vi "Select Physical Channels_Variable.vi"(8 "error in":errorcluster, 11 "Physical Channels In":bool[](array[boolean])) -> (0 "error out":errorcluster, 2 "Cancelled?":bool, 3 "Physical Channels Out":bool[](array[boolean]))   [LabVIEW 2020, in "Waveform Analog Output System Explorer.lvlib"]
doc: "When called, launches a dialogue to select AO channels to be added to the system definition"
uses:
  Waveform Analog Output System Explorer.lvlib
panel:
  in  "Tree":string(tree)
  in  "Cancel":bool
  in  "Accept":bool
  # "Please Select the Channels to Use"
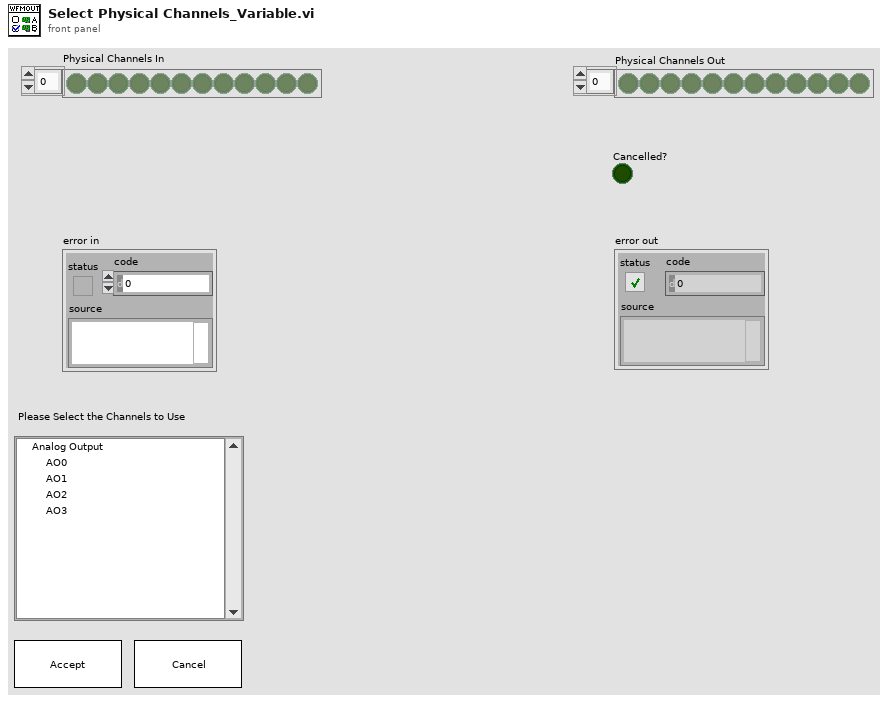
[diagram p1: front panel]
types:
  T1 = typedef "LVPoint32TypeDef.ctl" = cluster{"Horizontal":i32, "Vertical":i32}
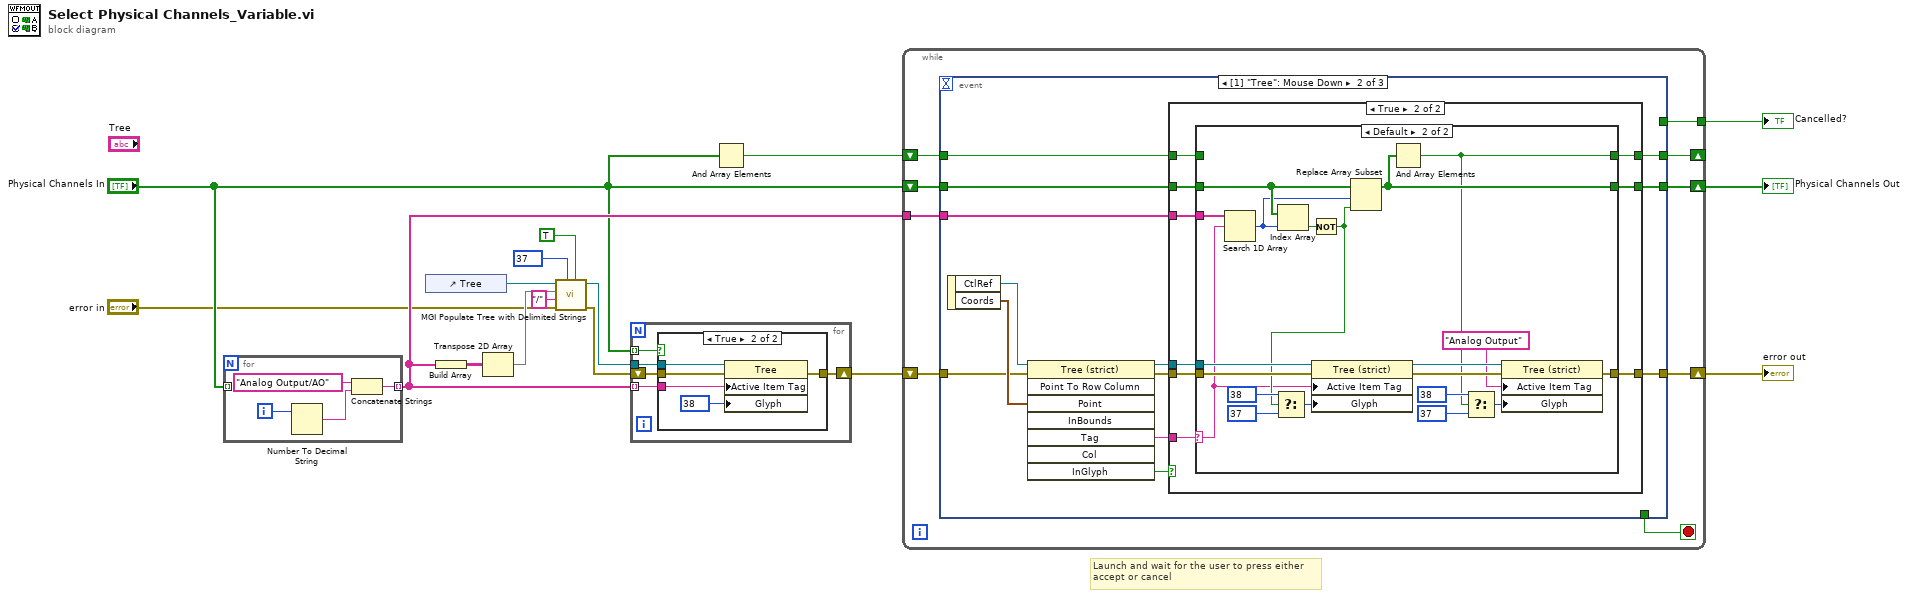
[diagram p0: block diagram]
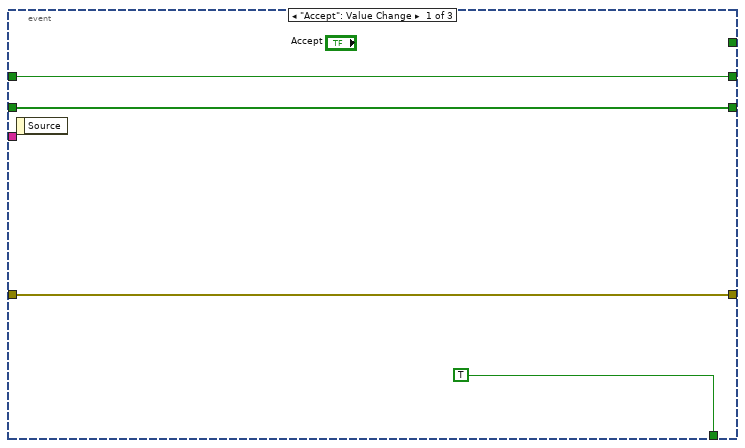
[diagram p3: hidden frame]
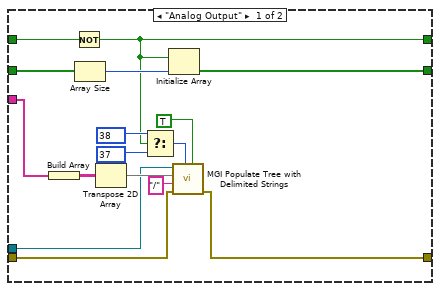
[diagram p5: hidden frame]
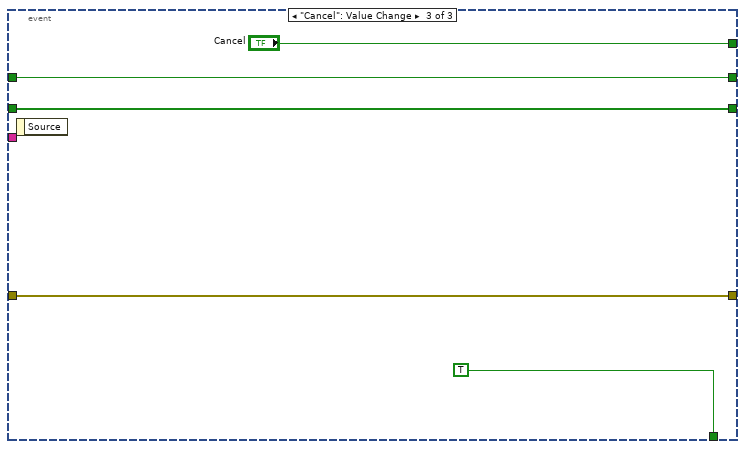
[diagram p6: hidden frame]
diagram:
  # "Launch and wait for the user to press either\naccept or cancel"
  n1 = for {
    tunnel: [w17] -> w5 mode=indexing
    tunnel: "Physical Channels In" -> [_] mode=indexing
    i -> [w20]
    n2 = Number To Decimal String(number=w20) -> (decimal integer string=w19:string)  [unwired: 1 in]
    n3 = Concatenate Strings("Analog Output/AO" ("string"), w19) -> (w17:string)
  }
  n4 = control-ref of="Tree"() -> (w14:refnum<vi>)
  n5 = Build Array(w5) -> (w11:string[][])
  n6 = Transpose 2D Array(2D array=w11) -> (transposed array=w9:string[][])
  n7 = call <userlib>:"MGI Populate Tree with Delimited Strings.vi"("Use Child Only?"=TRUE, "Default Symbol"=37, "error in (no error)"="error in", "Delimiter"="/", "Items (Delimited)"=w9, "Tree Control"=w14) -> ("error out"=w7:errorcluster, "Tree Control Dup"=w8:refnum<vi>)  [unwired: 3 in, 1 out]
  n8 = for {
    tunnel: w5 -> [w24] mode=indexing
    tunnel: "Physical Channels In" -> [w23] mode=indexing
    shift-right: [w21] -> w6
    shift-left: w7 -> [w22]
    tunnel: w8 -> [w25]
    n9 = case shown="True" w23 {
      tunnel: w25 -> [_ w31]
      tunnel: w24 -> [_ w30]
      tunnel: w22 -> [w26 w28]
      tunnel: [w26 w27] -> w21
      frame False {
      }
      frame True {
        n10 = property class="Tree"(reference=w31, error in=w28, "Active Item Tag"=w30, "Glyph"=38) -> (error out=w27:errorcluster)  [unwired: 1 out]
      }
    }
  }
  n11 = And Array Elements(Boolean array="Physical Channels In") -> (logical AND=w3:bool)
  n12 = while {
    tunnel: [w39] -> w15
    shift-right: [w40] -> w16
    shift-left: "Physical Channels In" -> [w38]
    shift-right: [w35] -> w4
    shift-left: w6 -> [w36]
    tunnel: w5 -> [w34]
    shift-right: [w32] -> _
    shift-left: w3 -> [w33]
    stop <- w37 stop-if-true
    n13 = event shown="[1] \"Tree\": Mouse Down" {
      selector: _ -> [_ _ _]
      dyn-events: _ -> [_ _ _]
      timeout: _ -> [_ _ _]
      tunnel: [w42 w52 w110] -> w40
      tunnel: w38 -> [w42 w51 w110]
      tunnel: [_ _ "Cancel"] -> w39
      tunnel: [TRUE _ TRUE] -> w37
      tunnel: w36 -> [w43 w54 w107]
      tunnel: [w43 w50 w107] -> w35
      tunnel: w34 -> [_ w48 _]
      tunnel: w33 -> [w41 w47 w106]
      tunnel: [w41 w46 w106] -> w32
      event "Accept": Value Change {
        n14 = event-data() -> ()  [unwired: 1 in, 1 out]
      }
      event "Tree": Mouse Down {
        n15 = event-data() -> ("CtlRef"=w45:refnum<vi>, "Coords"=w57:T1)  [unwired: 1 in]
        n16 = invoke class="Tree (strict)" method="Point To Row Column"(reference=w45, error in=w54, "Point"=w57) -> (reference out=w56:refnum<vi>, error out=w53:errorcluster, "Tag"=w55:string, "InGlyph"=w49:bool)  [unwired: 5 in, 4 out]
        n17 = case shown="True" w49 {
          tunnel: w56 -> [_ w69]
          tunnel: w55 -> [_ w63]
          tunnel: w53 -> [w59 w68]
          tunnel: [w60 w65] -> w52
          tunnel: w51 -> [w60 w64]
          tunnel: [w59 w67] -> w50
          tunnel: w48 -> [_ w66]
          tunnel: w47 -> [w58 w62]
          tunnel: [w58 w61] -> w46
          frame False {
          }
          frame True {
            n18 = case shown="Default" w63 {
              selector: w63 -> [_ w95]
              tunnel: w69 -> [w70 w105]
              tunnel: w68 -> [w72 w104]
              tunnel: [w71 w87] -> w67
              tunnel: w66 -> [w73 w103]
              tunnel: [w82 w94] -> w65
              tunnel: w64 -> [w84 w102]
              tunnel: w62 -> [w85 _]
              tunnel: [w79 w88] -> w61
              frame "Analog Output" {
                n19 = Build Array(w73) -> (w76:string[][])
                n20 = Not(x=w85) -> (.not. x?=w79:bool)
                n21 = Array Size(array=w84) -> (size(s)=w83:i32)
                n22 = Transpose 2D Array(2D array=w76) -> (transposed array=w78:string[][])
                n23 = Select(t=38, s=w79, f=37) -> (s? t:f=w74:i32)
                n24 = Initialize Array(w79, w83) -> (w82:bool[])
                n25 = call <userlib>:"MGI Populate Tree with Delimited Strings.vi"("Use Child Only?"=TRUE, "Default Symbol"=w74, "error in (no error)"=w72, "Delimiter"="/", "Items (Delimited)"=w78, "Tree Control"=w70) -> ("error out"=w71:errorcluster)  [unwired: 3 in, 2 out]
              }
              frame Default {
                n26 = Search 1D Array(1D array=w103, element=w95) -> (index of element=w100:i32)  [unwired: 1 in]
                n27 = Index Array(array=w102, index=w100) -> (element=w101:bool)
                n28 = Not(x=w101) -> (.not. x?=w96:bool)
                n29 = Select(t=38, s=w96, f=37) -> (s? t:f=w97:i32)
                n30 = property class="Tree (strict)"(reference=w105, error in=w104, "Active Item Tag"=w95, "Glyph"=w97) -> (reference out=w90:refnum<vi>, error out=w89:errorcluster)
                n31 = Replace Array Subset(array=w102, new element=w96, index=w100) -> (w94:bool[])
                n32 = And Array Elements(Boolean array=w94) -> (logical AND=w88:bool)
                n33 = Select(t=38, s=w88, f=37) -> (s? t:f=w93:i32)
                n34 = property class="Tree (strict)"(reference=w90, error in=w89, "Active Item Tag"="Analog Output" ("Active Item:Tag"), "Glyph"=w93) -> (error out=w87:errorcluster)  [unwired: 1 out]
              }
            }
          }
        }
      }
      event "Cancel": Value Change {
        n35 = event-data() -> ()  [unwired: 1 in, 1 out]
      }
    }
  }
  "Physical Channels Out" <- w16
  "Cancelled?" <- w15
  "error out" <- w4
